vi "Extract Error Call Chain.vi"(6 "Delete Call Chain?":bool, 8 "Error In":errorcluster) -> (0 "Error Out":errorcluster, 1 "Read Call Chain":string, 2 "Special Tag":string, 3 "Source":string)   [LabVIEW 2019, in "Error.lvclass"]
uses:
  Error.lvclass
  <vilib>/Utility/error.llb/TagReturnType.ctl
  3ade44d6-8e34-44bd-9993-33176f9b5ec5.vi
  <vilib>/Utility/Data Type/Get Numeric Information.vi
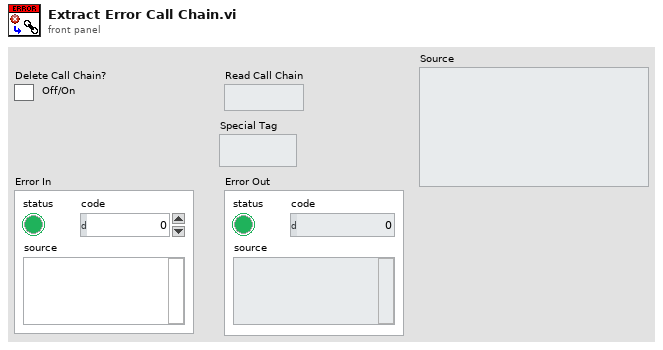
[diagram p1: front panel]
types:
  T1 = typedef "TagReturnType.ctl" = enum16{"No Tag", "<err>", "<append>"}
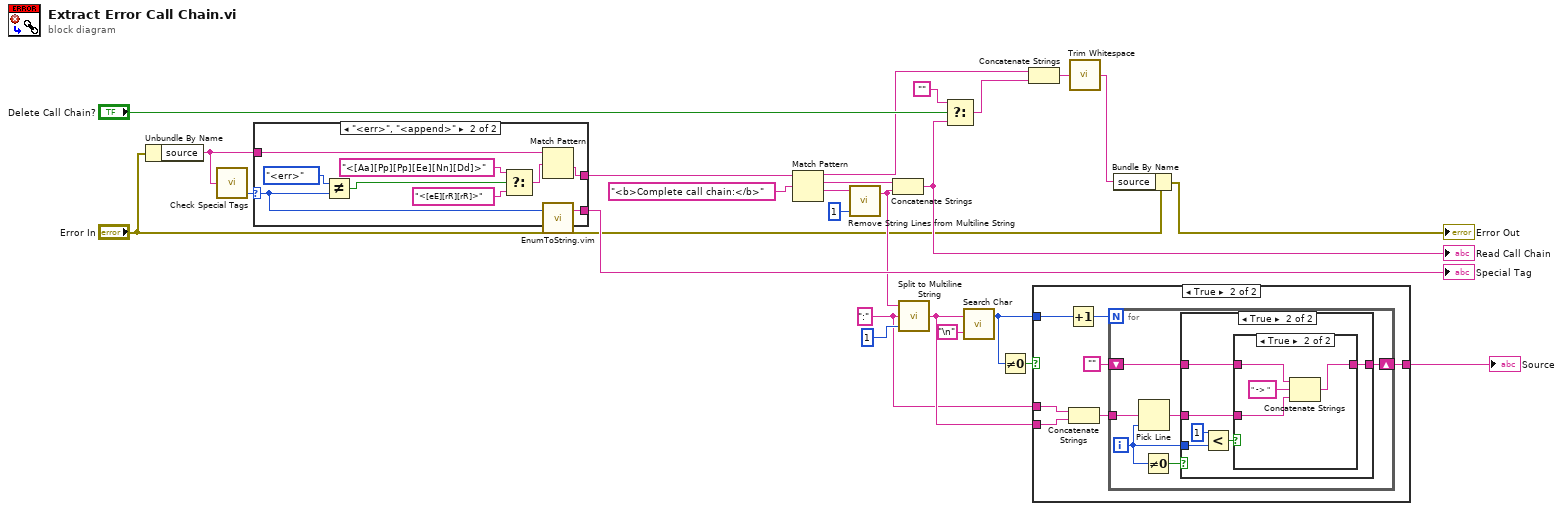
[diagram p0: block diagram]
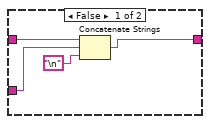
[diagram p3: hidden frame]
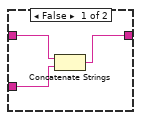
[diagram p4: hidden frame]
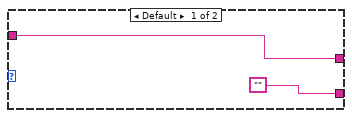
[diagram p5: hidden frame]
diagram:
  w1 = ":" ("delimiter")
  n1 = Unbundle By Name("Error In") -> ("source"=w17:string)
  n2 = call <vilib>:"Check Special Tags.vi"("source"=w17) -> ("Tag Found?"=w18:T1)  [unwired: 2 out]
  n3 = case shown="\"<err>\", \"<append>\"" w18 {
    selector: w18 -> [_ w33]
    tunnel: [w27 w36] -> w20
    tunnel: w17 -> [w27 w35]
    tunnel: ["" w34] -> w16
    frame Default {
    }
    frame "<err>", "<append>" {
      n4 = Not Equal?(x=TagReturnType."<err>", y=w33) -> (x != y?=w31:bool)
      n5 = Select(t="<[Aa][Pp][Pp][Ee][Nn][Dd]>" ("don't translate!"), s=w31, f="<[eE][rR][rR]>") -> (s? t:f=w30:string)
      n6 = Match Pattern(string=w35, regular expression=w30) -> (after substring=w36:string)  [unwired: 1 in, 3 out]
      n7 = call "EnumToString.vim"("Enum"=w33) -> ("Enum Value"=w34:string)  [unwired: 16 in, 2 out]
    }
  }
  "Special Tag" <- w16
  n8 = Match Pattern(string=w20, regular expression="<b>Complete call chain:</b>") -> (before substring=w15:string, match substring=w22:string, after substring=w10:string)  [unwired: 1 in, 1 out]
  n9 = call "Remove String Lines from Multiline String.vi"("Start Index (0)"=1 ("Lenght (1)"), "Multiline String"=w10) -> ("Output String"=w9:string)  [unwired: 1 in, 1 out]
  n10 = Concatenate Strings(w22, w9) -> (w23:string)
  "Read Call Chain" <- w23
  n11 = call "Split to Multiline String.vi"("Line Index"=1 ("line index"), "Delimiter"=w1, "Singleline String"=w9) -> ("Multiline String"=w6:string)
  n12 = Select(t="", s="Delete Call Chain?", f=w23) -> (s? t:f=w14:string)
  n13 = call "Search Char.vi"("Search Char"="\n", "Multiline String"=w6) -> ("Number of Char Found"=w4:i32)  [unwired: 1 out]
  n14 = Not Equal To 0?(x=w4) -> (x != 0?=w3:bool)
  n15 = Concatenate Strings(w15, w14) -> (w13:string)
  n16 = case shown="True" w3 {
    tunnel: w4 -> [_ w44]
    tunnel: w6 -> [w37 w42]
    tunnel: [w37 w40] -> w5
    tunnel: w1 -> [_ w38]
    frame False {
    }
    frame True {
      n17 = Increment(x=w44) -> (x+1=w43:i32)
      n18 = Concatenate Strings(w38, w42) -> (w39:string)
      n19 = for {
        N: w43 -> [_]
        tunnel: w39 -> [w50]
        shift-right: [w45] -> w40
        shift-left: "" -> [w46]
        i -> [w48]
        n20 = Pick Line(multi-line string=w50, line index=w48) -> (output string=w47:string)  [unwired: 1 in]
        n21 = Not Equal To 0?(x=w48) -> (x != 0?=w49:bool)
        n22 = case shown="True" w49 {
          tunnel: w48 -> [_ w60]
          tunnel: w47 -> [w52 w56]
          tunnel: [w53 w55] -> w45
          tunnel: w46 -> [w54 w57]
          frame False {
            n23 = Concatenate Strings(w54, w52, "\n") -> (w53:string)
          }
          frame True {
            n24 = Less?(x=1, y=w60) -> (x < y?=w59:bool)
            n25 = case shown="True" w59 {
              tunnel: w57 -> [w63 w67]
              tunnel: w56 -> [w62 w65]
              tunnel: [w61 w66] -> w55
              frame False {
                n26 = Concatenate Strings(w63, w62) -> (w61:string)
              }
              frame True {
                n27 = Concatenate Strings(w67, " -> " ("string"), w65) -> (w66:string)
              }
            }
          }
        }
      }
    }
  }
  "Source" <- w5
  n28 = call <vilib>:"Trim Whitespace.vi"("string"=w13) -> ("trimmed string"=w12:string)  [unwired: 1 in]
  n29 = Bundle By Name(cluster="Error In", "source"=w12) -> (→"Error Out":errorcluster)
